vi "Xsens Sample Counter (SubVI).vi"(1 "DATA In (Hex Display)":string) -> (0 "Sample Counter":u16)   [LabVIEW 2019]
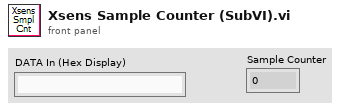
[diagram p1: front panel]
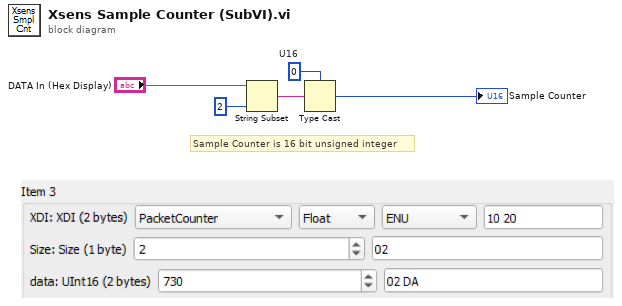
[diagram p0: block diagram]
diagram:
  w2 = u16 0  # U16
  # "Sample Counter is 16 bit unsigned integer"
  n1 = String Subset(string="DATA In (Hex Display)", length (rest)=2 ("length (rest)")) -> (substring=w3:string)  [unwired: 1 in]
  n2 = Type Cast(type=w2, x=w3) -> (*(type *) &x=→"Sample Counter":u16)
